vi "HandleRightClickMenuOption.vi"(0 "reference":refnum<class "Graph.lvclass">, 1 "MenuOption":string, 2 "graphics":refnum<class "Graphics.lvclass">, 3 "grid":refnum<class "Grid.lvclass">, 4 "point2D":T1 {"y" format="%.2f"; "x" format="%.2f"}, 5 "error in (no error)":errorcluster) -> (14 "reference out":refnum<class "Graph.lvclass">, 15 "Cancel":bool, 19 "error out":errorcluster)   [LabVIEW 2014, in "Graph.lvclass"]
doc: "HandleRightClickMenuOption"
uses:
  <resource>/Framework/Providers/Open_GDS/UML/Graph_class/Graph.lvclass
  <resource>/Framework/Providers/Open_GDS/UML/Graphics_class/Graphics.lvclass
  <resource>/Framework/Providers/Open_GDS/UML/Grid_class/Grid.lvclass
  <resource>/Framework/Providers/Open_GDS/UML/General/Point/Point Point2D.ctl
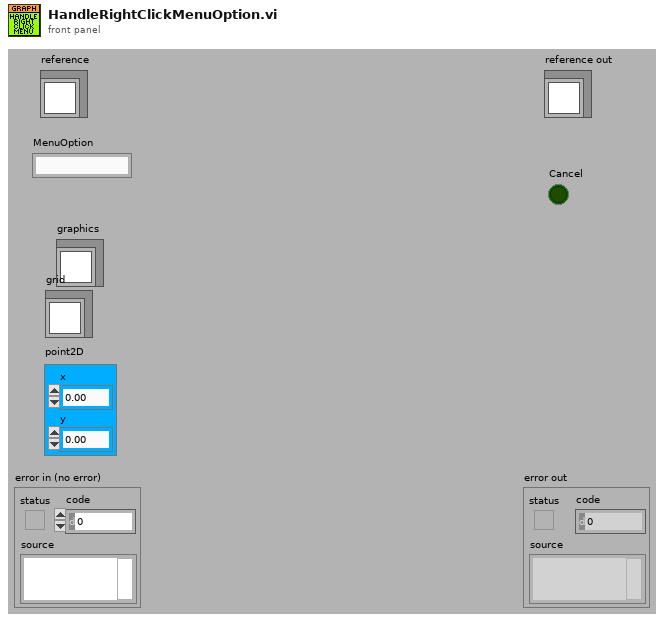
[diagram p1: front panel]
types:
  T1 = typedef "Point Point2D.ctl" = cluster{"x":dbl, "y":dbl}
  T2 = typedef "Graph.lvclass/ObjectAttributes.ctl" = cluster{"nodes":refnum<class "AbstractNode.lvclass">[], "edges":refnum<class "AbstractEdge.lvclass">[], "nodesToBeRemoved":refnum<class "AbstractNode.lvclass">[], "edgesToBeRemoved":refnum<class "AbstractEdge.lvclass">[], "needsLayout":bool, "LayoutNodes":refnum<class "AbstractNode.lvclass">[]}
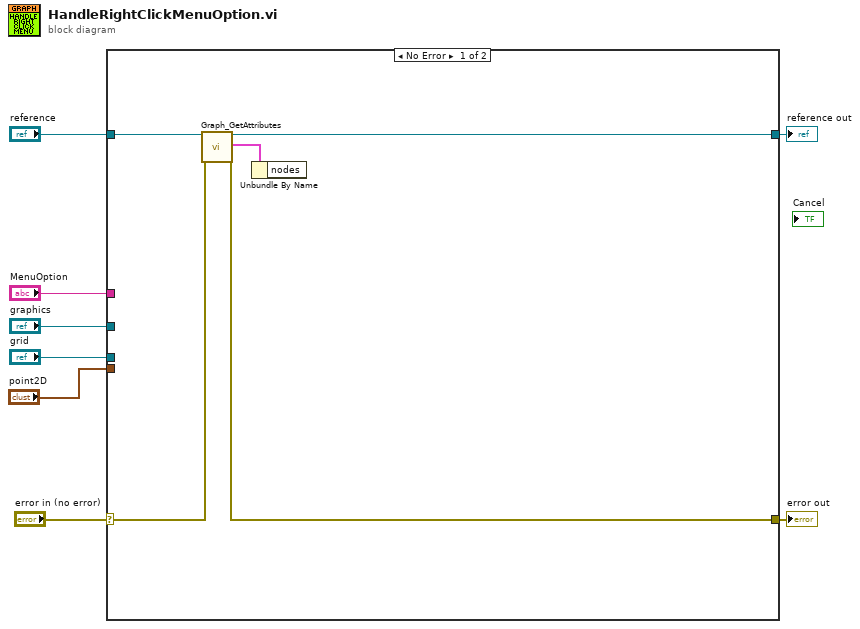
[diagram p0: block diagram]
diagram:
  n1 = case shown="No Error" "error in (no error)" {
    selector: "error in (no error)" -> [w10 w14]
    tunnel: "reference" -> [w13 w15]
    tunnel: [w12 w14] -> w7
    tunnel: [w11 w15] -> w6
    tunnel: "MenuOption" -> [_ _]
    tunnel: "graphics" -> [_ _]
    tunnel: "grid" -> [_ _]
    tunnel: "point2D" -> [_ _]
    frame No Error {
      n2 = call <resource>:"Graph_GetAttributes.vi"("reference in"=w13, "error in (no error)"=w10) -> ("reference out"=w11:refnum<class "Graph.lvclass">, "Data"=w9:T2, "error out"=w12:errorcluster)  [unwired: 1 in, 14 out]
      n3 = Unbundle By Name(w9) -> ()  [unwired: 1 out]
    }
    frame Error {
    }
  }
  "reference out" <- w6
  "error out" <- w7
